vi "DataView Test.vi"() -> ()   [LabVIEW 2013]
uses:
  SubVI/GVSMain Sub Window Global.vi
  DataView/VIEW/GVSNew View Global.vi
panel:
  in  "Add Bottom":bool
  in  "Add Top":bool
  in  "Add Right":bool
  in  "Add Left":bool
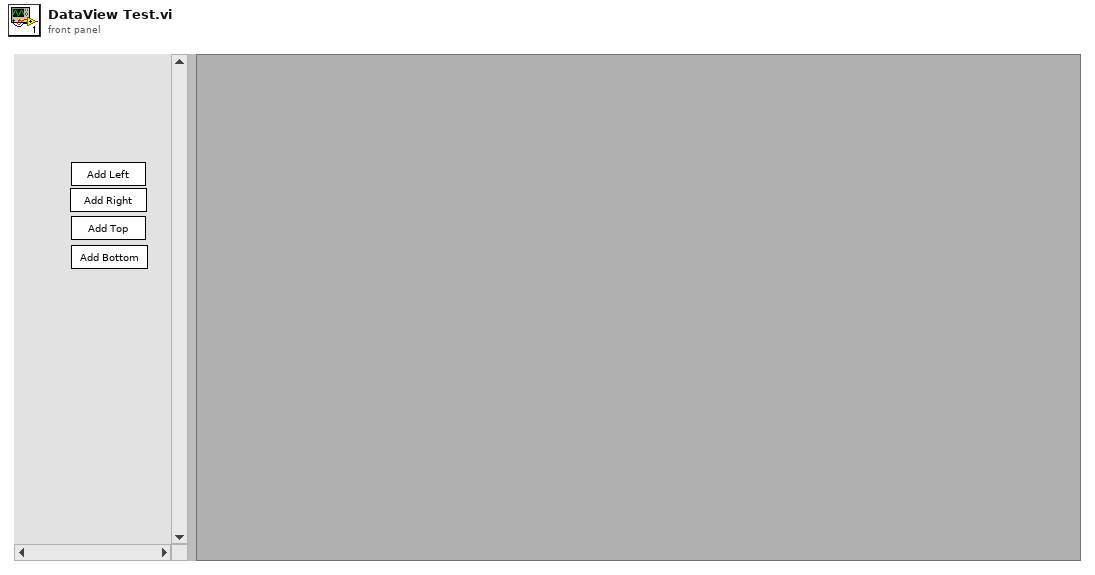
[diagram p1: front panel]
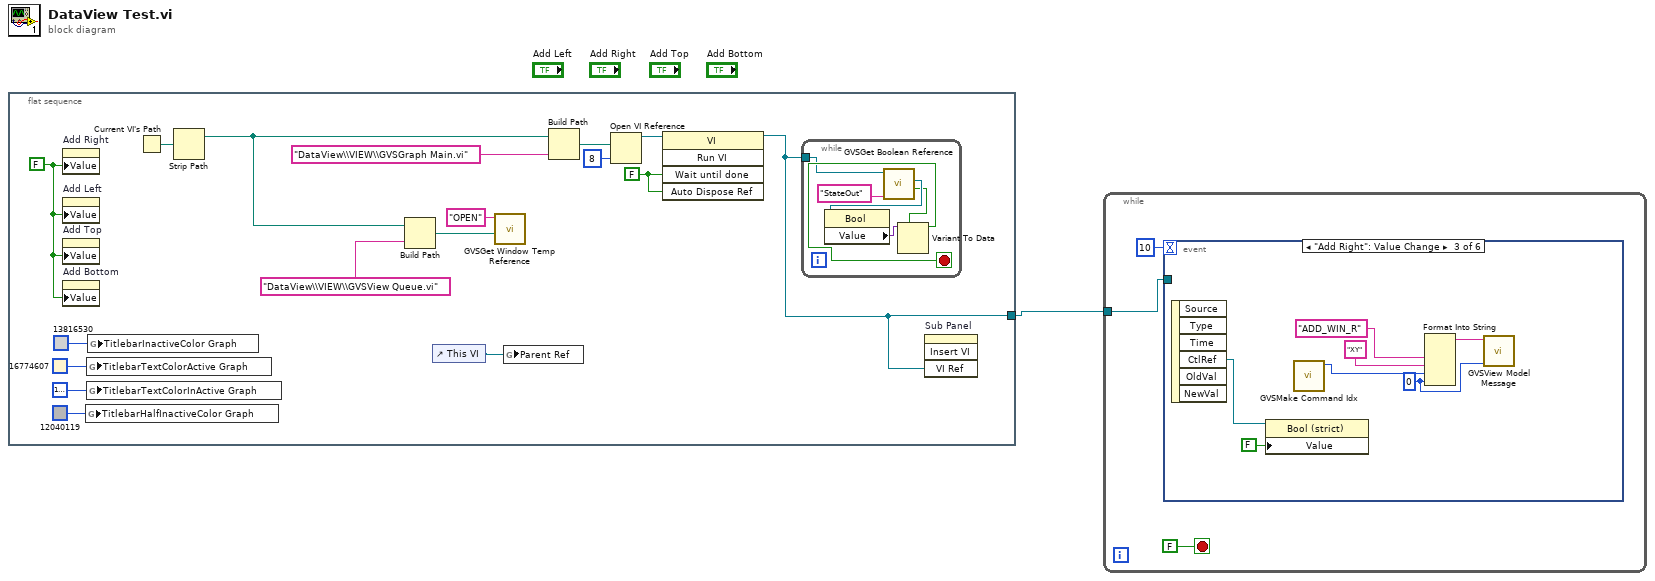
[diagram p0: block diagram]
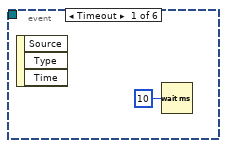
[diagram p2: hidden frame]
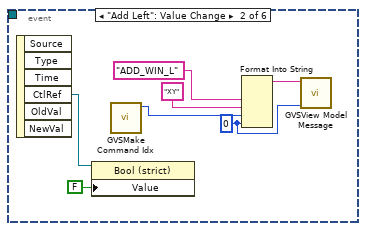
[diagram p3: hidden frame]
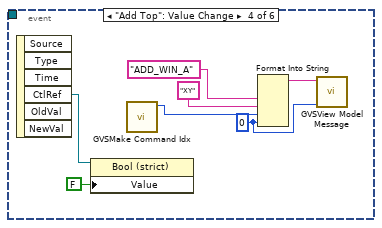
[diagram p4: hidden frame]
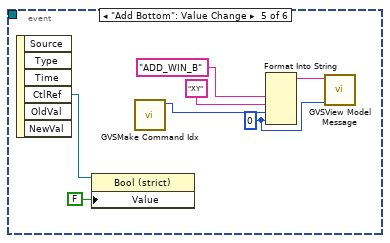
[diagram p5: hidden frame]
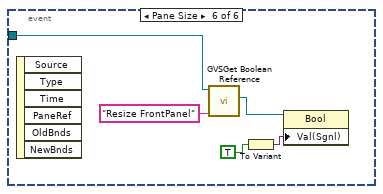
[diagram p6: hidden frame]
diagram:
  n1 = flat-sequence {
    tunnel: [w6] -> w1
    frame #0 {
      w13 = FALSE
      w7 = FALSE ("Wait Until Done")
      n2 = property on="Add Right" class="Bool (strict)"("Value"=w13) -> ()  [unwired: 2 in, 2 out]
      n3 = property on="Add Left" class="Bool (strict)"("Value"=w13) -> ()  [unwired: 2 in, 2 out]
      n4 = property on="Add Top" class="Bool (strict)"("Value"=w13) -> ()  [unwired: 2 in, 2 out]
      n5 = property on="Add Bottom" class="Bool (strict)"("Value"=w13) -> ()  [unwired: 2 in, 2 out]
      n6 = global write "GVSMain Sub Window Global.vi" "TitlebarHalfInactiveColor Graph"(u32 12040119 ("TitlebarHalfInActive")) -> ()
      n7 = global write "GVSMain Sub Window Global.vi" "TitlebarTextColorActive Graph"(u32 16774607 ("TextColorActive")) -> ()
      n8 = global write "GVSMain Sub Window Global.vi" "TitlebarTextColorInActive Graph"(u32 16777222 ("TextColorInActive")) -> ()
      n9 = global write "GVSMain Sub Window Global.vi" "TitlebarInactiveColor Graph"(u32 13816530 ("TitlebarInActive")) -> ()
      n10 = Current VI's Path() -> (path=w14:path)
      n11 = Strip Path(path=w14) -> (stripped path=w10:path)  [unwired: 1 out]
      n12 = Build Path(base path=w10, name or relative path="DataView\\VIEW\\GVSView Queue.vi") -> (appended path=w8:path)
      n13 = control-ref of="This VI"() -> (w12:refnum<vi>)
      n14 = call "GVSGet Window Temp Reference.vi"("sVIFullName"=w8, "sAction"="OPEN") -> ()  [unwired: 5 in, 5 out]
      n15 = global write "GVSNew View Global.vi" "Parent Ref"(w12) -> ()
      n16 = Build Path(base path=w10, name or relative path="DataView\\VIEW\\GVSGraph Main.vi") -> (appended path=w16:path)
      n17 = Open VI Reference(vi path=w16, options=8) -> (vi reference=w18:refnum<vi>)  [unwired: 4 in, 1 out]
      n18 = invoke class="VI" method="Run VI"(reference=w18, "Wait until done"=w7, "Auto Dispose Ref"=w7) -> (reference out=w6:refnum<vi>)  [unwired: 2 in, 4 out]
      n19 = while {
        tunnel: w6 -> [w19]
        stop <- w20 stop-if-true
        n20 = call "GVSGet Boolean Reference.vi"("Label Name"="StateOut", "VI Refnum"=w19) -> ("Boolean"=w21:bool, "Boolean Ref"=w23:refnum<vi>)  [unwired: 7 in, 1 out]
        n21 = property class="Bool"(reference=w23) -> ("Value"=w22:variant)  [unwired: 1 in, 2 out]
        n22 = Variant To Data(type=w21, Variant=w22) -> (data=w20:bool)  [unwired: 1 in, 1 out]
      }
      n23 = invoke on="Sub Panel" class="SubPanel" method="Insert VI"("VI Ref"=w6) -> ()  [unwired: 3 in, 4 out]
    }
  }
  n24 = while {
    tunnel: w1 -> [w25]
    stop <- FALSE stop-if-true
    n25 = event shown="[2] \"Add Right\": Value Change" {
      selector: _ -> [_ _ _ _ _ _]
      dyn-events: _ -> [_ _ _ _ _ _]
      timeout: 10 -> [_ _ _ _ _ _]
      tunnel: w25 -> [_ _ _ _ _ w61]
      event Timeout {
        n26 = event-data() -> ()  [unwired: 1 in, 3 out]
        n27 = Wait (ms)(milliseconds to wait=u32 10) -> ()  [unwired: 1 out]
      }
      event "Add Left": Value Change {
        w31 = 0 ("input 4")
        n28 = event-data() -> ("CtlRef"=w29:refnum<vi>)  [unwired: 1 in, 5 out]
        n29 = property class="Bool (strict)"(reference=w29, "Value"=FALSE) -> ()  [unwired: 1 in, 2 out]
        n30 = call "GVSMake Command Idx.vi"() -> ("New Command Idx"=w33:i32)  [unwired: 11 in]
        n31 = Format Into String("ADD_WIN_L" ("input 1"), "XY" ("input 2"), w33, w31) -> (resulting string=w32:string)  [unwired: 3 in, 1 out]
        n32 = call "GVSView Model Message.vi"("nData"=w31, "sMsgData"=w32) -> ()  [unwired: 7 in, 3 out]
      }
      event "Add Right": Value Change {
        w38 = 0 ("input 4")
        n33 = event-data() -> ("CtlRef"=w36:refnum<vi>)  [unwired: 1 in, 5 out]
        n34 = property class="Bool (strict)"(reference=w36, "Value"=FALSE) -> ()  [unwired: 1 in, 2 out]
        n35 = call "GVSMake Command Idx.vi"() -> ("New Command Idx"=w40:i32)  [unwired: 11 in]
        n36 = Format Into String("ADD_WIN_R" ("input 1"), "XY" ("input 2"), w40, w38) -> (resulting string=w39:string)  [unwired: 3 in, 1 out]
        n37 = call "GVSView Model Message.vi"("nData"=w38, "sMsgData"=w39) -> ()  [unwired: 7 in, 3 out]
      }
      event "Add Top": Value Change {
        w45 = 0 ("input 4")
        n38 = event-data() -> ("CtlRef"=w44:refnum<vi>)  [unwired: 1 in, 5 out]
        n39 = property class="Bool (strict)"(reference=w44, "Value"=FALSE) -> ()  [unwired: 1 in, 2 out]
        n40 = call "GVSMake Command Idx.vi"() -> ("New Command Idx"=w47:i32)  [unwired: 11 in]
        n41 = Format Into String("ADD_WIN_A" ("input 1"), "XY" ("input 2"), w47, w45) -> (resulting string=w46:string)  [unwired: 3 in, 1 out]
        n42 = call "GVSView Model Message.vi"("nData"=w45, "sMsgData"=w46) -> ()  [unwired: 7 in, 3 out]
      }
      event "Add Bottom": Value Change {
        w52 = 0 ("input 4")
        n43 = event-data() -> ("CtlRef"=w50:refnum<vi>)  [unwired: 1 in, 5 out]
        n44 = property class="Bool (strict)"(reference=w50, "Value"=FALSE) -> ()  [unwired: 1 in, 2 out]
        n45 = call "GVSMake Command Idx.vi"() -> ("New Command Idx"=w54:i32)  [unwired: 11 in]
        n46 = Format Into String("ADD_WIN_B" ("input 1"), "XY" ("input 2"), w54, w52) -> (resulting string=w53:string)  [unwired: 3 in, 1 out]
        n47 = call "GVSView Model Message.vi"("nData"=w52, "sMsgData"=w53) -> ()  [unwired: 7 in, 3 out]
      }
      event Pane Size {
        n48 = event-data() -> ()  [unwired: 1 in, 6 out]
        n49 = call "GVSGet Boolean Reference.vi"("Label Name"="Resize FrontPanel", "VI Refnum"=w61) -> ("Boolean Ref"=w59:refnum<vi>)  [unwired: 7 in, 2 out]
        n50 = To Variant(anything=TRUE) -> (Variant=w58:variant)
        n51 = property class="Bool"(reference=w59, "Val(Sgnl)"=w58) -> ()  [unwired: 1 in, 2 out]
      }
    }
  }
